vi "Untitled2 (SubVI).vi"(10 "channels":string, 11 "IVI Refnum in":refnum<k15>) -> (1 "String":string, 2 "Array":string[](array[string]), 3 "IVI Refnum out":refnum<k15>)   [LabVIEW 2011, in "PXIDigitizer.lvclass"]
uses:
  PXIDigitizer.lvclass
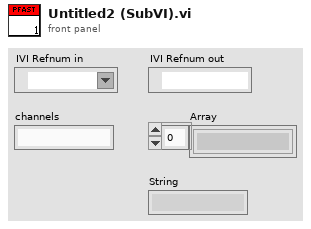
[diagram p1: front panel]
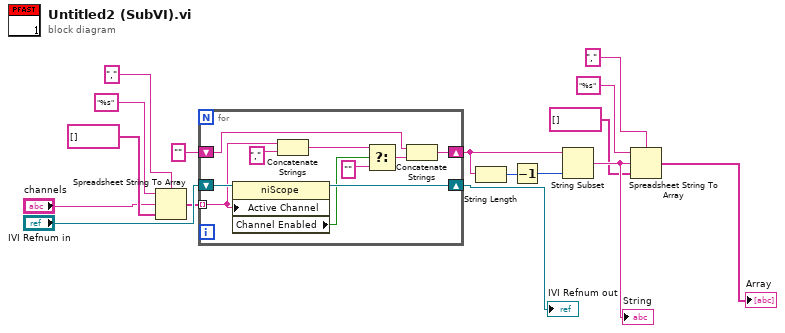
[diagram p0: block diagram]
diagram:
  n1 = Spreadsheet String To Array(delimiter (Tab)=",", format string="%s", spreadsheet string="channels", array type (2D Dbl)=string[] []) -> (array=w9:string[])
  n2 = for {
    shift-right: [w25] -> w13
    shift-left: "IVI Refnum in" -> [w26]
    tunnel: w9 -> [w21] mode=indexing
    shift-right: [w18] -> w14
    shift-left: "" -> [w17]
    n3 = property class="niScope"(reference=w26, "Active Channel"=w21) -> (reference out=w25:refnum<k15>, "Channel Enabled"=w24:bool)  [unwired: 1 in, 1 out]
    n4 = Concatenate Strings(w21, "," ("string")) -> (w20:string)
    n5 = Select(t=w20, s=w24, f="") -> (s? t:f=w19:string)
    n6 = Concatenate Strings(w17, w19) -> (w18:string)
  }
  "IVI Refnum out" <- w13
  n7 = String Length(string=w14) -> (length=w11:i32)
  n8 = Decrement(x=w11) -> (x-1=w12:i32)
  n9 = String Subset(string=w14, length (rest)=w12) -> (substring=w15:string)  [unwired: 1 in]
  "String" <- w15
  n10 = Spreadsheet String To Array(delimiter (Tab)=",", format string="%s", spreadsheet string=w15, array type (2D Dbl)=string[] []) -> (array=→"Array":string[])
